vi "ChangePolarity_Kiethley2614_B.vi"(1 "Voltage (sourse)":dbl) -> ()   [LabVIEW 2017]
panel:
  in  "GPIB Address":string="12"
  in  "error in (no error)":errorcluster
  out "error out":errorcluster
  # "Channel B"
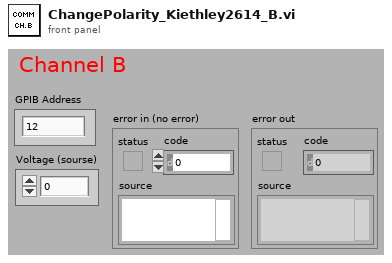
[diagram p1: front panel]
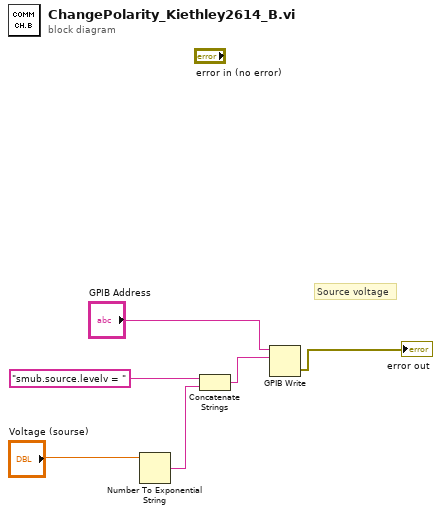
[diagram p0: block diagram]
diagram:
  # "Source voltage"
  n1 = Number To Exponential String(number="Voltage (sourse)") -> (E-format string=w4:string)  [unwired: 3 in]
  n2 = Concatenate Strings("smub.source.levelv = ", w4) -> (w3:string)
  n3 = GPIB Write(0:"GPIB Address", 1:w3) -> (6:→"error out":errorcluster)  [unwired: 3 in, 1 out]
